vi "find Relative VS Ref.vi"(7 "Relative Type":u16(ring) items=["Targets", "Controller", "Custom Devices", "This CD", "This CD/Group", "This CD/Group/SubGroup"], 8 "error in (no error)":errorcluster, 11 "Item Ref in":T1 format="%.0x") -> (0 "error out":errorcluster, 1 "Item Path out":string, 2 "Relative Item Ref Out":T1 format="%.0x", 3 "Item Ref out":T1 format="%.0x", 4 "Found":bool)   [LabVIEW 2016, in "FPGA Resource Manager System Definition.lvlib"]
uses:
  FPGA Resource Manager System Definition.lvlib
  <vilib>/NI Veristand/Custom Device API/Custom Device Item Ref.ctl
  NationalInstruments.VeriStand.SystemStorage
  <vilib>/NI VeriStand/Custom Device API/Custom Device API.lvlib
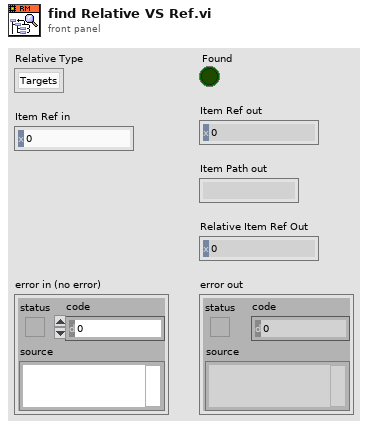
[diagram p1: front panel]
types:
  T1 = typedef "Custom Device API.lvlib/Custom Device Item Ref.ctl" = u64
  T2 = typedef "Custom Device API.lvlib/Custom Device Pointer.ctl" = refnum<k24>
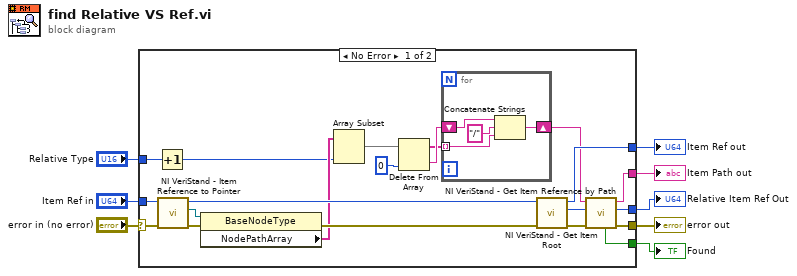
[diagram p0: block diagram]
diagram:
  n1 = case shown="No Error" "error in (no error)" {
    selector: "error in (no error)" -> [w18 w34]
    tunnel: [w29 _] -> w1
    tunnel: [w28 w35] -> w2
    tunnel: [w24 _] -> w3
    tunnel: "Item Ref in" -> [w19 w35]
    tunnel: "Relative Type" -> [w15 _]
    tunnel: [w17 w34] -> w7
    tunnel: [w13 _] -> w8
    frame No Error {
      n2 = Increment(x=w15) -> (x+1=w16:u16)
      n3 = call <vilib>:"NI VeriStand - Item Reference to Pointer.vi"("error in (no error)"=w18, "Item Ref in"=w19) -> ("error out"=w25:errorcluster, "Node Pointer"=w20:T2, "Item Ref out"=w22:T1)  [unwired: 6 in, 1 out]
      n4 = property class="BaseNodeType"(reference=w20, error in=w25) -> (error out=w26:errorcluster, "NodePathArray"=w21:string[])  [unwired: 1 out]
      n5 = Array Subset(array=w21, length=w16) -> (w12:string[])  [unwired: 1 in]
      n6 = Delete From Array(array=w12, index=0) -> (deleted portion=w11:string, array with subset deleted=w10:string[])  [unwired: 1 in]
      n7 = for {
        tunnel: w10 -> [w32] mode=indexing
        shift-right: [w30] -> w23
        shift-left: w11 -> [w31]
        n8 = Concatenate Strings(w31, "/" ("string"), w32) -> (w30:string)
      }
      n9 = call <vilib>:"NI VeriStand - Get Item Root.vi"("error in (no error)"=w26, "Item Ref in"=w22) -> ("error out"=w27:errorcluster, "Root Ref out"=w14:T1, "Item Ref out"=w28:T1)  [unwired: 6 in, 1 out]
      n10 = call <vilib>:"NI VeriStand - Get Item Reference by Path.vi"("error in (no error)"=w27, "Root Ref"=w14, "Item Path in"=w23) -> ("error out"=w17:errorcluster, "Item Ref"=w29:T1, "Item Path out"=w24:string, "Found"=w13:bool)  [unwired: 5 in]
    }
    frame Error {
    }
  }
  "Relative Item Ref Out" <- w1
  "Item Ref out" <- w2
  "Item Path out" <- w3
  "error out" <- w7
  "Found" <- w8
